vi "Sum_of_Two_Dice.vi"() -> ()   [LabVIEW 2025]
uses:
  <vilib>/numeric/Random Number (Range) U64.vi
  <vilib>/numeric/sub_Random U32.vi
panel:
  out "Dice 1+2":dbl
  out "Dice 2":dbl
  out "Dice 1":u64
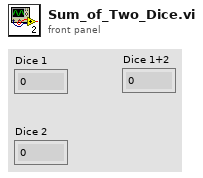
[diagram p1: front panel]
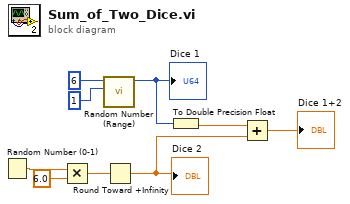
[diagram p0: block diagram]
diagram:
  n1 = Random Number (0-1)() -> (number: 0 to 1=w7:dbl)
  n2 = Multiply(x=w7, y=6.0) -> (x*y=w5:dbl)
  n3 = call-poly <vilib>:"Random Number (Range).vi"("lower bound (0)"=u64 1, "upper bound (100)"=u64 6) -> ("number"=w4:u64)  [unwired: 9 in]
  "Dice 1" <- w4
  n4 = Round Toward +Infinity(x=w5) -> (ceil(x): smallest int >= x=w1:dbl)
  "Dice 2" <- w1
  n5 = To Double Precision Float(number=w4) -> (double precision float=w3:dbl)
  n6 = Add(x=w3, y=w1) -> (x+y=→"Dice 1+2":dbl)
